vi "sampleexcitjob.vi"(0 "sample port":refnum<visa-resource-name>[](array[refnum]), 2 "sample sn":string[](array[string])) -> (7 "Array":bool[](array[boolean]), 8 "error":errorcluster[](array[cluster]))   [LabVIEW 2012]
uses:
  globalstatus.vi
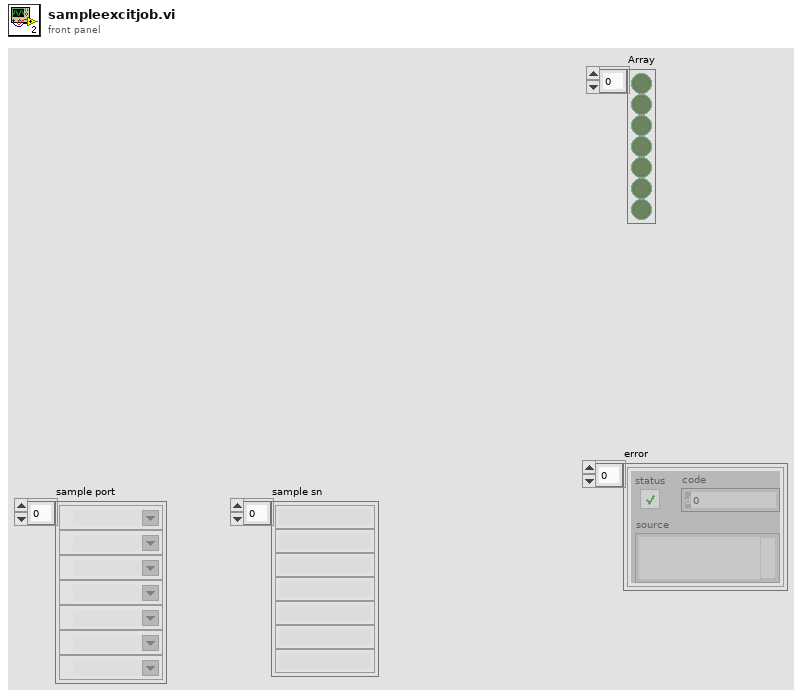
[diagram p1: front panel]
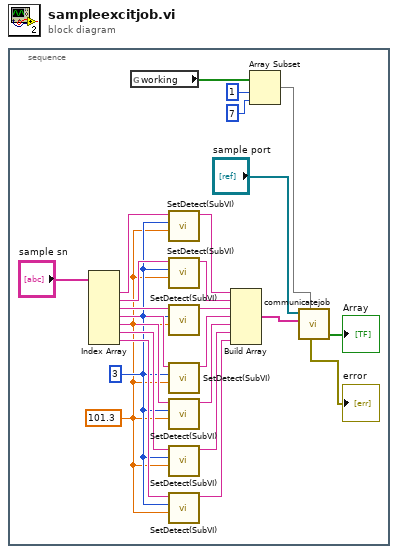
[diagram p0: block diagram]
diagram:
  n1 = stacked-sequence {
    frame #0 {
      w14 = 101.3
      w15 = 3
      n2 = Index Array(array="sample sn") -> (element #1=w24:string, element #2=w23:string, element #3=w22:string, element #4=w21:string, element #5=w20:string, element #6=w19:string, element #7=w16:string)  [unwired: 7 in]
      n3 = global read "globalstatus.vi" "working"() -> (w3:bool[])
      n4 = call "SetDetect(SubVI).vi"("pressure"=w14, "led selected"=w15, "sn"=w24) -> ("output frame"=w11:string)  [unwired: 8 in]
      n5 = call "SetDetect(SubVI).vi"("pressure"=w14, "led selected"=w15, "sn"=w23) -> ("output frame"=w10:string)  [unwired: 8 in]
      n6 = call "SetDetect(SubVI).vi"("pressure"=w14, "led selected"=w15, "sn"=w22) -> ("output frame"=w9:string)  [unwired: 8 in]
      n7 = call "SetDetect(SubVI).vi"("pressure"=w14, "led selected"=w15, "sn"=w21) -> ("output frame"=w8:string)  [unwired: 8 in]
      n8 = call "SetDetect(SubVI).vi"("pressure"=w14, "led selected"=w15, "sn"=w20) -> ("output frame"=w5:string)  [unwired: 8 in]
      n9 = call "SetDetect(SubVI).vi"("pressure"=w14, "led selected"=w15, "sn"=w19) -> ("output frame"=w6:string)  [unwired: 8 in]
      n10 = call "SetDetect(SubVI).vi"("pressure"=w14, "led selected"=w15, "sn"=w16) -> ("output frame"=w7:string)  [unwired: 8 in]
      n11 = Build Array(w11, w10, w9, w8, w5, w6, w7) -> (w12:string[])
      n12 = Array Subset(array=w3, index=1, length=7) -> (w4:bool[])
      n13 = call "communicatejob.vi"("sample port"="sample port", "condition"=w4, "send command"=w12) -> ("error"=→"error":errorcluster[], "receive result"=→"Array":bool[])  [unwired: 2 in, 2 out]
    }
  }
